vi "Initialise Raw Data Stream Reader.vi"(8 "error in (no error)":errorcluster, 11 "IP Address":string) -> (0 "error out":errorcluster={"status"=TRUE, "code"=-314004, "source"="Create Network Stream Reader Endpoint in Initialise Spectrum Reader.vi->Host_Main.vi"}, 3 "reader endpoint":refnum<k21>)   [LabVIEW 2016]
uses:
  <vilib>/dex/Stream Element Allocation Mode.ctl
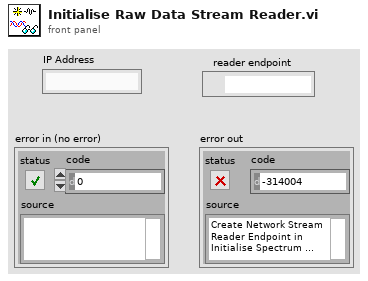
[diagram p1: front panel]
types:
  T1 = typedef "Stream Element Allocation Mode.ctl" = u32
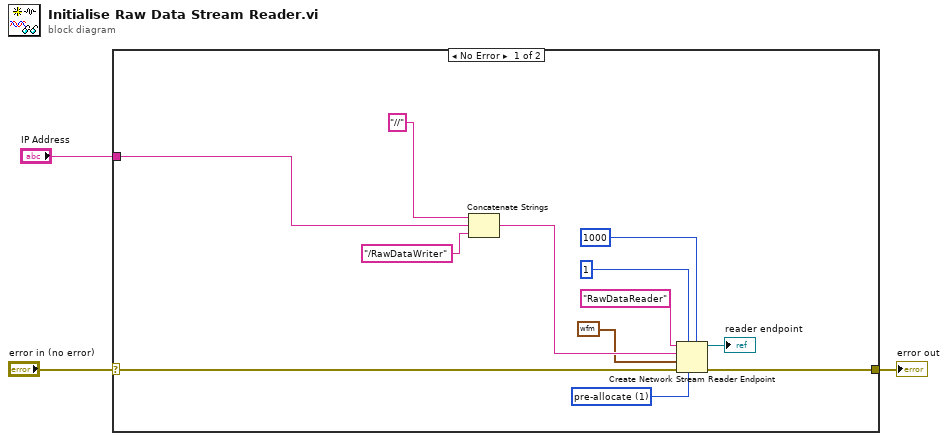
[diagram p0: block diagram]
diagram:
  n1 = case shown="No Error" "error in (no error)" {
    selector: "error in (no error)" -> [w9 w16]
    tunnel: [w14 w16] -> w3
    tunnel: "IP Address" -> [w4 _]
    frame No Error {
      w6 = T1 1 items=["allocate as needed", "pre-allocate"] ("element allocation mode")
      n2 = Concatenate Strings("//", w4, "/RawDataWriter" ("string")) -> (w10:string)
      n3 = Create Network Stream Reader Endpoint(5:1000 ("timeout in ms (-1)"), 6:w6, 7:1 ("reader buffer size"), 8:w9, 9:waveform(u8) {"t0"=timestamp(0 s since 1904-01-01), "dt"=1.0, "Y"=[]} ("output waveform"), 10:w10, 11:"RawDataReader" ("reader name")) -> (0:w14:errorcluster, 3:→"reader endpoint":refnum<k21>)
    }
    frame Error {
    }
  }
  "error out" <- w3
